vi "LongToByteArr.vi"(1 "CANET 端口":u32) -> (0 "Array":u8[](array[numeric]))   [LabVIEW 2014]
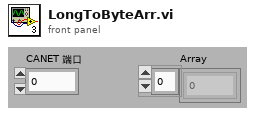
[diagram p1: front panel]
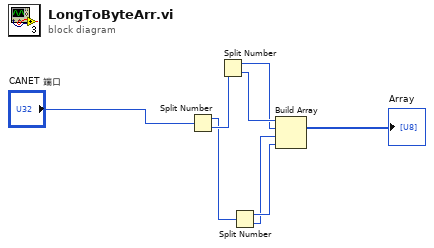
[diagram p0: block diagram]
diagram:
  n1 = Split Number(x="CANET 端口") -> (hi(x)=w1:u16, lo(x)=w7:u16)
  n2 = Split Number(x=w7) -> (hi(x)=w4:u8, lo(x)=w5:u8)
  n3 = Split Number(x=w1) -> (hi(x)=w3:u8, lo(x)=w2:u8)
  n4 = Build Array(w5, w4, w2, w3) -> (→"Array":u8[])
